vi "Emit EOF.vi"(8 "error in (no error)":errorcluster, 11 "JSON Lexer in":refnum<class "JSON Lexer.lvclass">) -> (0 "error out":errorcluster, 3 "JSON Lexer out":refnum<class "JSON Lexer.lvclass">)   [LabVIEW 2019, in "JKI JSON Serialization.lvlib" / "JSON Lexer.lvclass"]
doc: "JKI JSON 1.1.10.37\nTomi Maila - JKI\nCopyright (c) 2017, JKI"
uses:
  JSON Lexer.lvclass
  JSON Token.ctl
  JSON Token Type.ctl
  JSON Lexer.lvclass/JSON Lexer.ctl
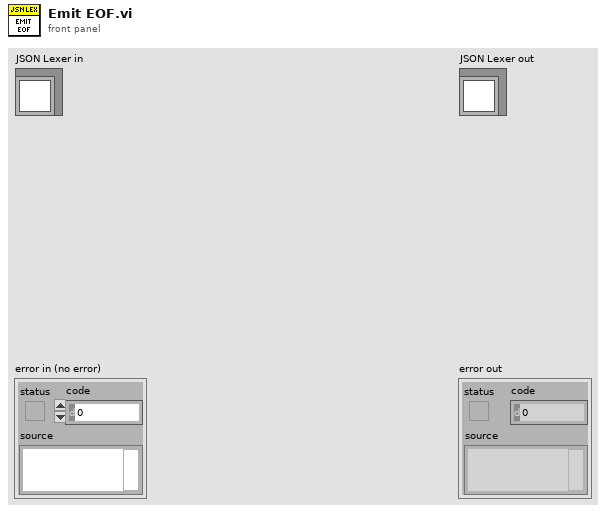
[diagram p1: front panel]
types:
  T1 = typedef "JKI JSON Serialization.lvlib/JSON Lexer.lvclass/JSON Token.ctl" = cluster{"Token Type":T2, "Token Value":string}
  T2 = typedef "JKI JSON Serialization.lvlib/JSON Lexer.lvclass/JSON Token Type.ctl" = enum32{"unknown", "comma", "end-label", "begin-object", "end-object", "begin-array", "end-array", "quoted-string", "boolean", "exponential-number", "decimal-number", "integer-number", "special-number", "null", "symbol", "whitespace", "EOF"}
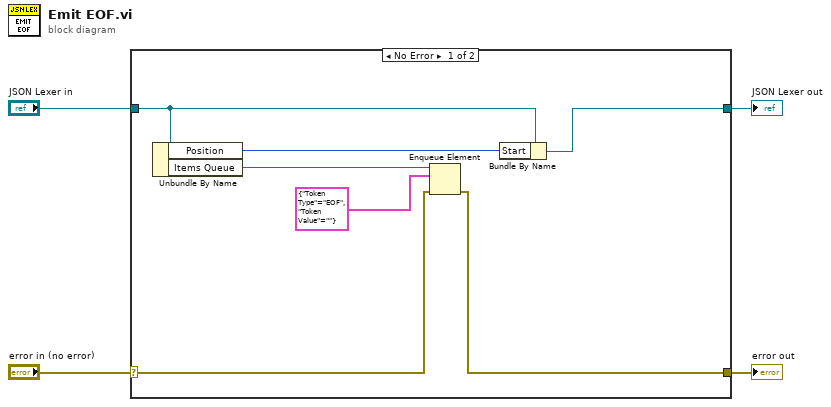
[diagram p0: block diagram]
diagram:
  n1 = case shown="No Error" "error in (no error)" {
    selector: "error in (no error)" -> [w8 w13]
    tunnel: [w7 w13] -> w3
    tunnel: [w10 w12] -> w1
    tunnel: "JSON Lexer in" -> [w11 w12]
    frame No Error {
      n2 = Unbundle By Name(w11) -> ("Position"=w6:i32, "Items Queue"=w9:refnum<queue>)
      n3 = Enqueue Element(queue=w9, element=T1 {"Token Type"=enum."EOF", "Token Value"=""}, error in (no error)=w8) -> (error out=w7:errorcluster)  [unwired: 1 in, 2 out]
      n4 = Bundle By Name(cluster=w11, "Start"=w6) -> (w10:refnum<class "JSON Lexer.lvclass">)
    }
    frame Error {
    }
  }
  "error out" <- w3
  "JSON Lexer out" <- w1
